vi "GetMeasEchoMaxEnab.vi"(8 "错误输入（无错误）":errorcluster, 11 "SelGateType":i32) -> (0 "错误输出":errorcluster, 3 "返回值":u8)   [LabVIEW 2014]
uses:
  ZXUTConfigMgr.dll
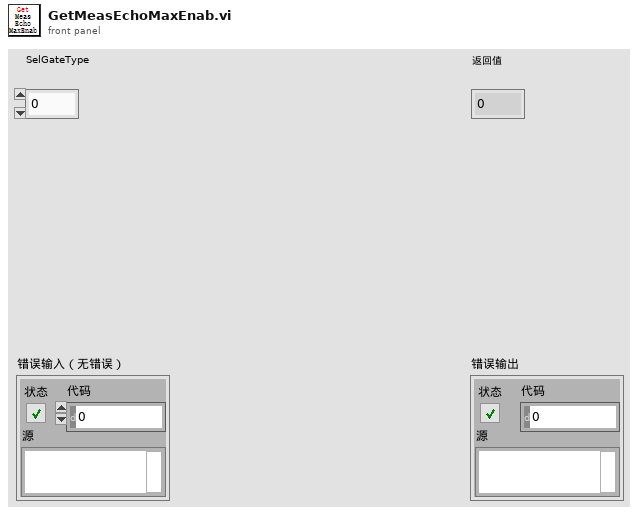
[diagram p1: front panel]
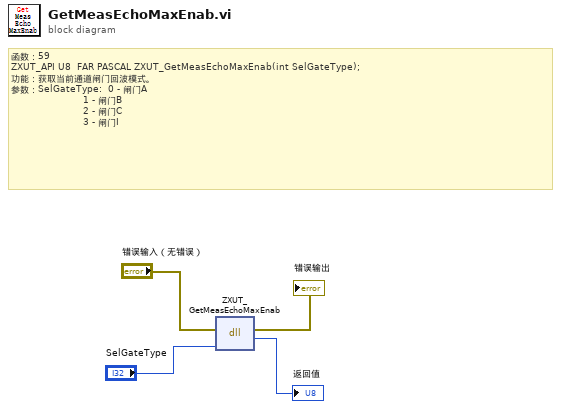
[diagram p0: block diagram]
diagram:
  # "函数：59\nZXUT_API U8\t\tFAR PASCAL ZXUT_GetMeasEchoMaxEnab(int SelGateType);\n功能：获取当前通道闸门回波模式。\n参数：SelGateType:  0 - 闸门A \n                        1 - 闸门B\n                        2 - 闸门C\n                        3 - 闸门I"
  n1 = dll-call lib="PTH2eabs D软件超声实时监测软件ZXUTAppDemo(华南理工V02.00)X86DllZXUTConfigMgr.dll" fn="ZXUT_GetMeasEchoMaxEnab"(error in="错误输入（无错误）", "SelGateType"="SelGateType") -> (error out=→"错误输出":errorcluster, "返回值"=→"返回值":u8)  [unwired: 3 in, 1 out]
